vi "ExFileReadNDisplayRGBInteractiveTif.vi"() -> ()   [LabVIEW 2010]
panel:
  in  "Set values":bool
  in  "TIF output":path=path "C:/Program Files/SIToolKit/LabVIEW/Data Files/test"
  out "Blue Offset read":dbl format="%.2f"
  out "Green Offset read":dbl format="%.2f"
  out "Red Offset read":dbl format="%.2f"
  out "Blue Gain read":dbl format="%.2f"
  out "Green Gain read":dbl format="%.2f"
  out "Red Gain read":dbl format="%.2f"
  in  "Blue Offset":dbl format="%.2f"
  in  "Green Offset":dbl format="%.2f"
  in  "Red Offset":dbl format="%.2f"
  in  "Blue Gain":dbl=1.0 format="%.2f"
  in  "Red Gain":dbl=1.0 format="%.2f"
  in  "Green Gain":dbl=1.0 format="%.2f"
  in  "Bit shift":u16
  in  "Type of Bayer":u32=1 max=4 step=1
  in  "Full File Name":path=path "C:/Program Files/SIToolKit/LabVIEW/Data Files/Color.SPE"
  in  "?":bool
  in  "FileType":u32=67371008
  out "error out":errorcluster
  in  "error in (no error)":errorcluster
  # "ExReadFileNDisplayRGBInteractiveTif.vi\nThis example will read in a file of the selected data type and display as RGB frame. When finished viewing data, make sure to use the STOP button to close the display. This example allows the gain, bit shift and offsets to be \nset interactively."
  # "File Types:\nSPE = 67371008\nTIF   = 67174400\nPMI  = 67436544"
  # "Browse match pattern is set to *.tif.  Modify this if different file type is needed."
  # "Interactive section"
  # "This will properly close\nthe image and\ndeallocate memory."
  # "NOTICE\n\nTHIS VI REQUIRES THAT THE TOOLKIT\nBE UNLOADED BY RUNNING THE\n VI EXCLOSEGLOBALCAM.VI\n BEFORE LEAVING LABVIEW."
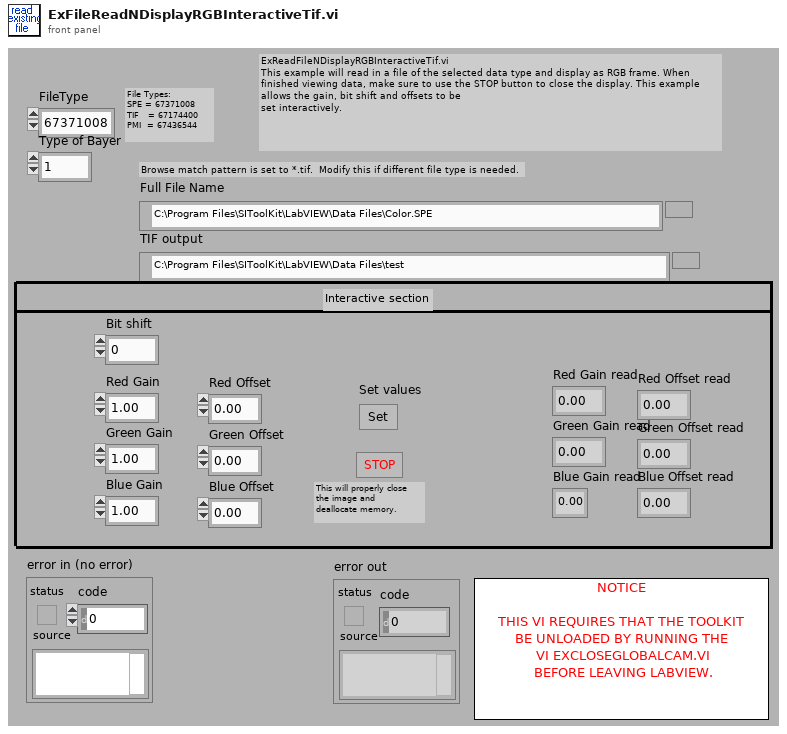
[diagram p1: front panel]
types:
  T1 = cluster{"Type of Bayer":u32, "Red Gain":dbl, "Green Gain":dbl, "Blue Gain":dbl, "Bit shift":u16, "Red Offset":dbl, "Green Offset":dbl, "Blue Offset":dbl}
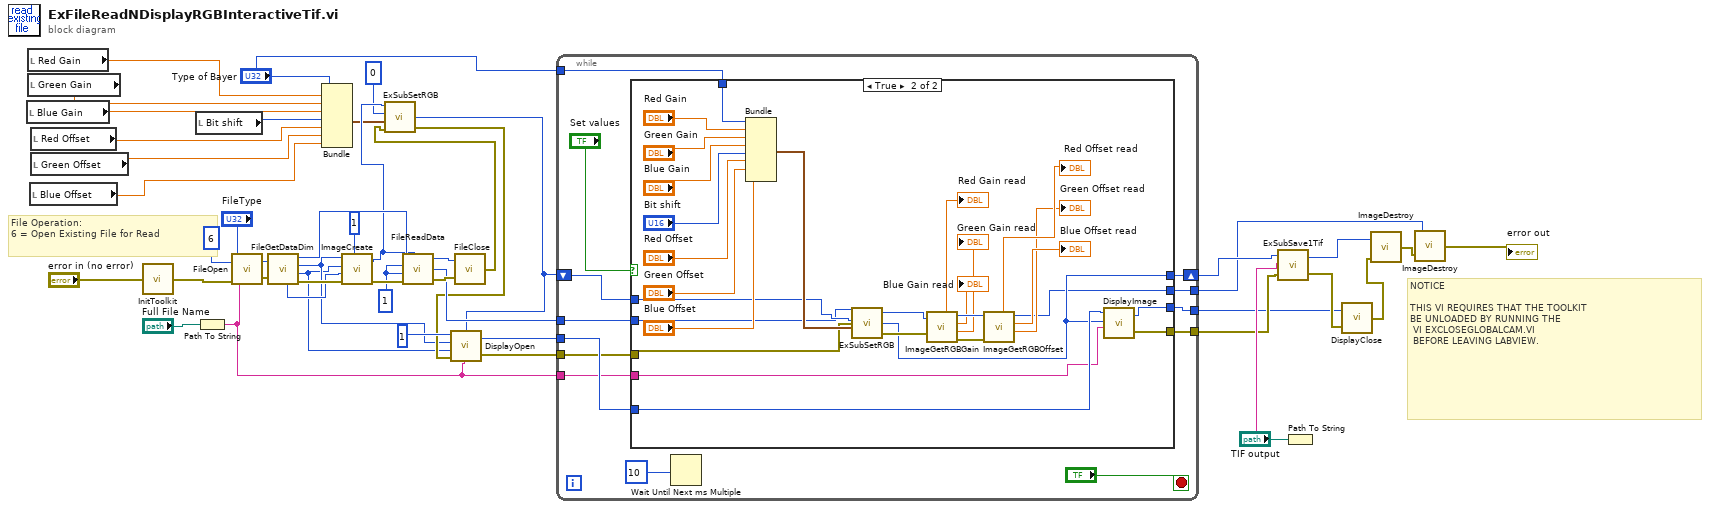
[diagram p0: block diagram]
diagram:
  w35 = 1
  # "NOTICE\n\nTHIS VI REQUIRES THAT THE TOOLKIT\nBE UNLOADED BY RUNNING THE\n VI EXCLOSEGLOBALCAM.VI\n BEFORE LEAVING LABVIEW."
  # "File Operation:\n6 = Open Existing File for Read"
  n1 = local read "Blue Gain"() -> (w6:dbl)
  n2 = local read "Red Gain"() -> (w8:dbl)
  n3 = local read "Green Gain"() -> (w7:dbl)
  n4 = local read "Blue Offset"() -> (w3:dbl)
  n5 = local read "Red Offset"() -> (w5:dbl)
  n6 = local read "Green Offset"() -> (w4:dbl)
  n7 = call <userlib>:"InitToolkit.vi"("error in"="error in (no error)") -> ("error out"=w45:errorcluster)
  n8 = local read "Bit shift"() -> (w9:u16)
  n9 = Path To String(path="Full File Name") -> (string=w26:string)
  n10 = call <userlib>:"FileOpen.vi"("error in"=w45, "File Operations"=u32 6 ("File Operation"), "FileName"=w26, "File Type"="FileType") -> ("error out"=w43:errorcluster, "File Handle"=w42:u32)
  n11 = call <userlib>:"FileGetDataDim.vi"("File Handle"=w42, "error in"=w43) -> ("Data Type"=w13:u32, "File Handle"=w37:u32, "X dim"=w12:u32, "Y dim"=w11:u32, "error out"=w41:errorcluster)  [unwired: 1 out]
  n12 = Bundle("Type of Bayer"="Type of Bayer", "Red Gain"=w8, "Green Gain"=w7, "Blue Gain"=w6, "Bit shift"=w9, "Red Offset"=w5, "Green Offset"=w4, "Blue Offset"=w3) -> (w2:T1)  [unwired: 1 in]
  n13 = call <userlib>:"ImageCreate.vi"("X dimension"=w12, "Y dimension"=w11, "Data Type"=w13, "error in"=w41, "Number Of Frames"=1) -> ("Image Handle"=w17:u32, "error out"=w36:errorcluster)
  n14 = call <userlib>:"FileReadData.vi"("File Handle"=w37, "Start Frame"=w35, "End Frame"=w35, "error in"=w36, "Image Handle"=w17) -> ("File Handle"=w31:u32, "Image Handle"=w27:u32, "error out"=w30:errorcluster)
  n15 = call <userlib>:"FileClose.vi"("error in"=w30, "File Handle"=w31) -> ("error out"=w14:errorcluster)
  n16 = call "ExSubSetRGB.vi"("error in (no error)"=w14, "Adjustments"=w2, "RGB Handle"=0, "Image handle"=w17) -> ("error out"=w15:errorcluster, "RGB handle"=w10:u32)  [unwired: 1 out]
  n17 = call <userlib>:"DisplayOpen.vi"("Display Title"=w26, "Image Handle"=w10, "error in"=w15, "Display Height"=w11, "Display Width"=w12, "Display Type"=1) -> ("error out"=w28:errorcluster, "Display Handle"=w29:u32)
  n18 = while {
    tunnel: [w60] -> w24
    tunnel: w29 -> [w57]
    tunnel: w28 -> [w56]
    tunnel: w27 -> [w55]
    tunnel: w26 -> [w54]
    tunnel: [w53] -> w25
    tunnel: "Type of Bayer" -> [w51]
    shift-right: [w49] -> w20
    shift-left: w10 -> [w50]
    tunnel: [w48] -> w18
    stop <- "?" stop-if-true
    n19 = case shown="True" "Set values" {
      tunnel: [w62 w92] -> w60
      tunnel: w57 -> [w62 w83]
      tunnel: w56 -> [w61 w71]
      tunnel: w55 -> [w63 w67]
      tunnel: w54 -> [_ w82]
      tunnel: [w61 w81] -> w53
      tunnel: w51 -> [_ w77]
      tunnel: w50 -> [w64 w68]
      tunnel: [w64 w66] -> w49
      tunnel: [w63 w65] -> w48
      frame False {
      }
      frame True {
        n20 = Bundle("Type of Bayer"=w77, "Red Gain"="Red Gain", "Green Gain"="Green Gain", "Blue Gain"="Blue Gain", "Bit shift"="Bit shift", "Red Offset"="Red Offset", "Green Offset"="Green Offset", "Blue Offset"="Blue Offset") -> (w72:T1)  [unwired: 1 in]
        n21 = call "ExSubSetRGB.vi"("error in (no error)"=w71, "Adjustments"=w72, "RGB Handle"=w68, "Image handle"=w67) -> ("error out"=w70:errorcluster, "RGB handle"=w66:u32, "Image handle"=w69:u32)
        n22 = call <userlib>:"ImageGetRGBGain.vi"("Image Handle"=w69, "error in (no error)"=w70) -> ("Red"=→"Red Gain read":dbl, "Image Handle"=w90:u32, "Blue"=→"Blue Gain read":dbl, "Green"=→"Green Gain read":dbl, "error out"=w91:errorcluster)  [unwired: 1 out]
        n23 = call <userlib>:"ImageGetRGBOffset.vi"("Image Handle"=w90, "error in (no error)"=w91) -> ("Red"=→"Red Offset read":dbl, "Image Handle"=w65:u32, "Blue"=→"Blue Offset read":dbl, "Green"=→"Green Offset read":dbl)  [unwired: 2 out]
        n24 = call <userlib>:"DisplayImage.vi"("Title"=w82, "Image Handle"=w66, "Display Handle"=w83) -> ("error out"=w81:errorcluster, "Display Handle"=w92:u32)  [unwired: 1 in]
      }
    }
    n25 = Wait Until Next ms Multiple(millisecond multiple=10) -> ()  [unwired: 1 out]
  }
  n26 = Path To String(path="TIF output") -> (string=w32:string)
  n27 = call "ExSubSave1Tif.vi"("error in (no error)"=w25, "File name"=w32, "Image Handle"=w20) -> ("error out"=w34:errorcluster, "Image handle"=w19:u32)
  n28 = call <userlib>:"DisplayClose.vi"("error in"=w34, "Display Handle"=w24) -> ("error out"=w22:errorcluster)
  n29 = call <userlib>:"ImageDestroy.vi"("error in"=w22, "Data handle"=w19) -> ("error out"=w21:errorcluster)
  n30 = call <userlib>:"ImageDestroy.vi"("error in"=w21, "Data handle"=w18) -> ("error out"=→"error out":errorcluster)
